vi "GetVideoOptionsCodes.vi"(8 "error in (no error)":errorcluster, 11 "CameraDemo in":refnum<class "CameraDemo.lvclass">) -> (0 "error out":errorcluster, 2 "VideoOptionsCodes":T1 {"ImageTypeCodesList"."Code" format="%.0x"; "VideoResolutionCodesList"."Code" format="%.0x"; "FrameRateCodesList"."Code" format="%.0x"}, 3 "CameraDemo out":refnum<class "CameraDemo.lvclass">)   [LabVIEW 2020, in "CameraI2COUSB.lvlib" / "CameraDemo.lvclass"]
uses:
  CameraDemo.lvclass
  ICamera/ICamera/TypeDef/VideoOptionsCodes.ctl
  CameraDemo.lvclass/CameraDemo.ctl
  ICamera/ICamera/ICamera.lvclass
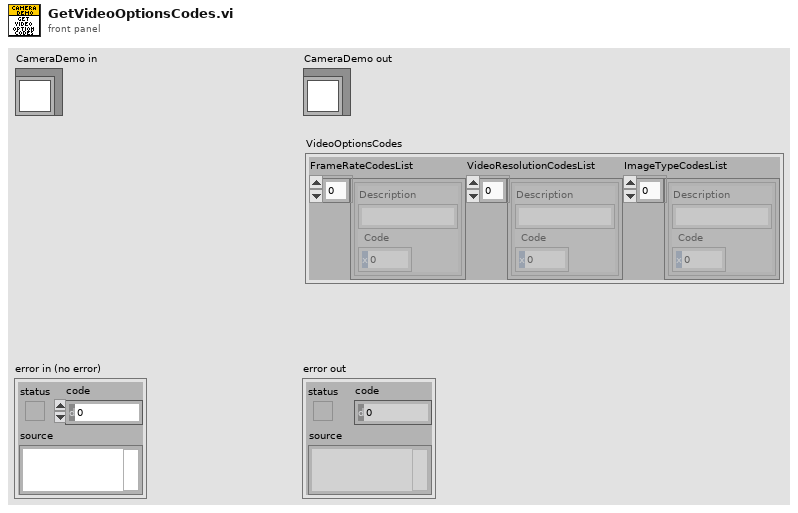
[diagram p1: front panel]
types:
  T1 = typedef "ICamera.lvlib/ICamera.lvclass/VideoOptionsCodes.ctl" = cluster{"FrameRateCodesList":cluster{"Description":string, "Code":u8}[], "VideoResolutionCodesList":cluster{"Description":string, "Code":u8}[], "ImageTypeCodesList":cluster{"Description":string, "Code":u8}[]}
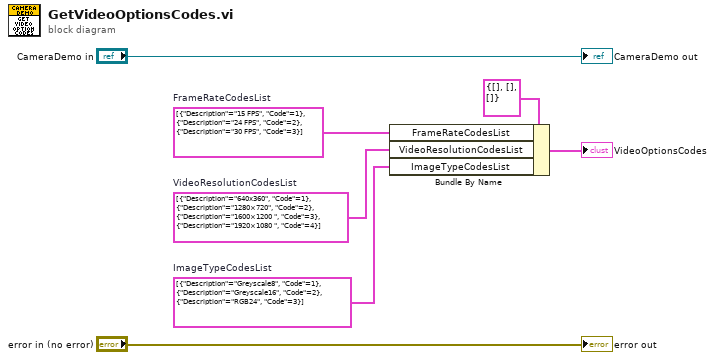
[diagram p0: block diagram]
diagram:
  w5 = cluster{"Description":string, "Code":u8}[] [{"Description"="Greyscale8", "Code"=1}, {"Description"="Greyscale16", "Code"=2}, {"Description"="RGB24", "Code"=3}]  # ImageTypeCodesList
  w1 = cluster{"Description":string, "Code":u8}[] [{"Description"="640x360", "Code"=1}, {"Description"="1280×720", "Code"=2}, {"Description"="1600×1200 ", "Code"=3}, {"Description"="1920×1080 ", "Code"=4}]  # VideoResolutionCodesList
  w2 = cluster{"Description":string, "Code":u8}[] [{"Description"="15 FPS", "Code"=1}, {"Description"="24 FPS", "Code"=2}, {"Description"="30 FPS", "Code"=3}]  # FrameRateCodesList
  n1 = Bundle By Name(cluster=T1 {"FrameRateCodesList"=[], "VideoResolutionCodesList"=[], "ImageTypeCodesList"=[]} ("VideoOptionsCodes"), "FrameRateCodesList"=w2, "VideoResolutionCodesList"=w1, "ImageTypeCodesList"=w5) -> (→"VideoOptionsCodes":T1)
  "error out" <- "error in (no error)"
  "CameraDemo out" <- "CameraDemo in"
